vi "SetSignalParams.vi"(8 "error in (no error)":errorcluster, 10 "Variant":variant, 11 "FunctionBase in":refnum<class "FunctionBase.lvclass">) -> (0 "error out":errorcluster, 3 "FunctionBase out":refnum<class "FunctionBase.lvclass">)   [LabVIEW 2018, in "Functions.lvlib" / "FunctionBase.lvclass"]
uses:
  FunctionBase.lvclass
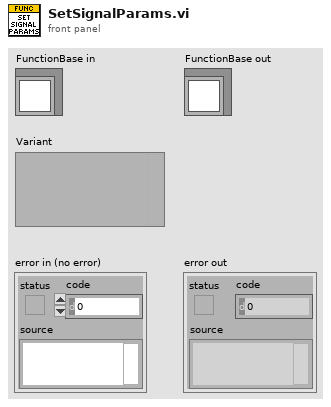
[diagram p1: front panel]
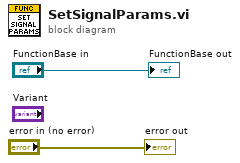
[diagram p0: block diagram]
diagram:
  "error out" <- "error in (no error)"
  "FunctionBase out" <- "FunctionBase in"
